vi "Twitter Open - Embedded.vi"(5 "Access Secret":string, 7 "Access Token":string, 8 "error in":errorcluster, 10 "Consumer Secret":string, 11 "Consumer Key":string) -> (0 "error out":errorcluster, 3 "Twitter Handle Out":T1={"OAuth Credentials"={"Signature Method"=enum."HMAC-SHA1", "Version"="1.0", "Client"={"Token"="", "Secret"=""}, "Access"={"Token"="", "Secret"=""}}, "since ID"="", "max ID"="", "Screen Name"=""})   [LabVIEW 2011, in "i3-twitter.lvlib"]
doc: "<b>Twitter Open - Embedded</b> is used when the application has a specific set of Access Credentials or the user is on a platform without a web browser.\n\nThe <b>Consumer Key</b> and <b>Consumer Secret</b> are unique to each application and can be created by making an application at dev.twitter.com. See the Twitter Getting Started Guide for more details.\n\nUse of this function requires <b>Access Credentials</b> which can be found on dev.twitter.com when an application is created or by using the <b>Twitter Open - Desktop VI</b> on a computer with a Web Browser to have the user grant access and create an Access Token and Access Secret for use on the embedded system."
uses:
  i3-twitter.lvlib
  Controls/Twitter Handle.ctl
  i3-oauth/Controls/OAuth Handle.ctl
  i3-oauth/Controls/Signature Method.ctl
  i3-oauth/Controls/Credentials.ctl
  i3-oauth/i3-oauth.lvlib
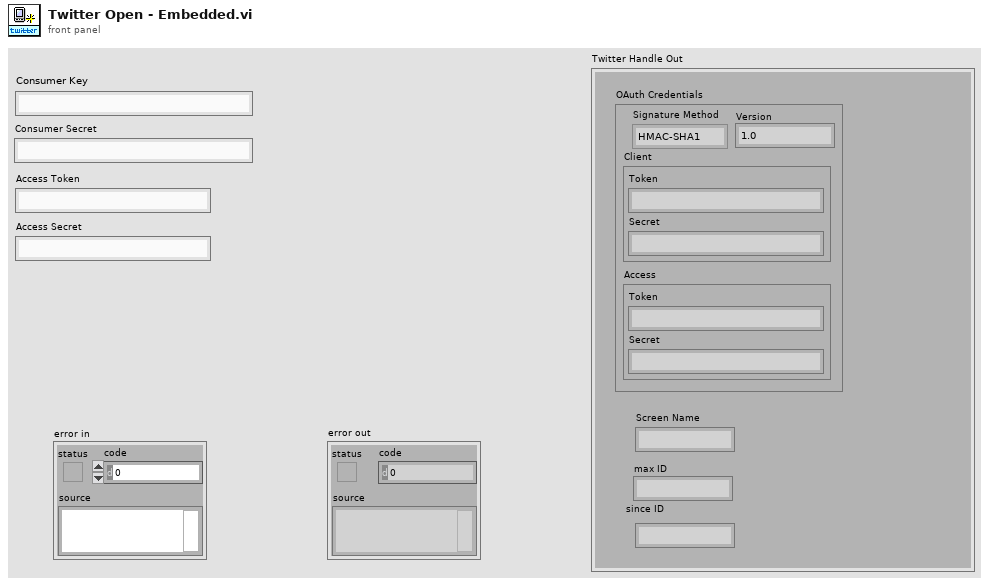
[diagram p1: front panel]
types:
  T1 = typedef "i3-twitter.lvlib/Twitter Handle.ctl" = cluster{"OAuth Credentials":T2, "since ID":string, "max ID":string, "Screen Name":string}
  T2 = typedef "i3-oauth.lvlib/OAuth Handle.ctl" = cluster{"Signature Method":T3, "Version":string, "Client":T4, "Access":T4}
  T3 = typedef "i3-oauth.lvlib/Signature Method.ctl" = enum16{"HMAC-MD5", "HMAC-SHA1", "HMAC-SHA224", "HMAC-SHA256", "HMAC-SHA384", "HMAC-SHA512"}
  T4 = typedef "i3-oauth.lvlib/Credentials.ctl" = cluster{"Token":string, "Secret":string}
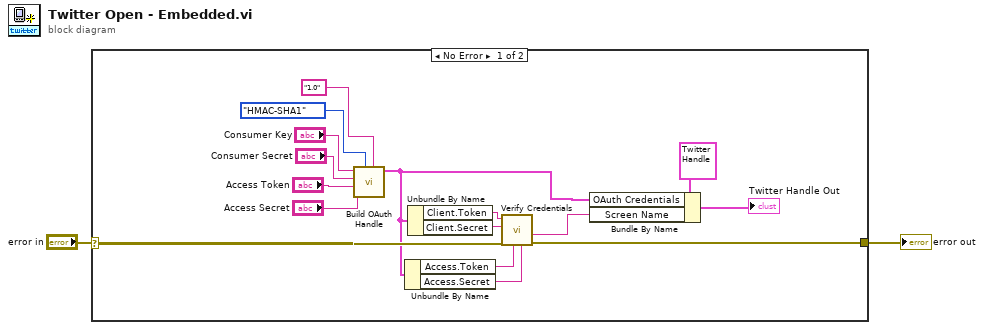
[diagram p0: block diagram]
diagram:
  n1 = case shown="No Error" "error in" {
    selector: "error in" -> [w14 w19]
    tunnel: [w17 w19] -> w2
    frame No Error {
      n2 = call "Build OAuth Handle.vi"("Version (1.0)"="1.0", "Signature Method (HMAC-SHA1)"=Signature_Method."HMAC-SHA1", "Access Secret"="Access Secret", "Access Token"="Access Token", "Client Secret"="Consumer Secret", "Client Token"="Consumer Key") -> ("OAuth Handle"=w5:T2)  [unwired: 5 in]
      n3 = Unbundle By Name(w5) -> ("Access.Token"=w7:string, "Access.Secret"=w6:string)
      n4 = Unbundle By Name(w5) -> ("Client.Token"=w8:string, "Client.Secret"=w9:string)
      n5 = call "Verify Credentials.vi"("Access Token Secret (In)"=w6, "Access Token (In)"=w7, "error in (no error)"=w14, "Consumer Secret"=w9, "Consumer Key"=w8) -> ("error out"=w17:errorcluster, "Screen Name"=w16:string)  [unwired: 3 in, 2 out]
      n6 = Bundle By Name(cluster=T1 {"OAuth Credentials"={"Signature Method"=enum."HMAC-MD5", "Version"="", "Client"={"Token"="", "Secret"=""}, "Access"={"Token"="", "Secret"=""}}, "since ID"="", "max ID"="", "Screen Name"=""} ("Twitter Handle"), "OAuth Credentials"=w5, "Screen Name"=w16) -> (→"Twitter Handle Out":T1)
    }
    frame Error {
    }
  }
  "error out" <- w2
